vi "AlliGator Set New ROI Name.vi"(2 "Stored ROIs in":T1[](array[typedef]) {"ROI Descriptor"."Contours"."Type" items=["No Selection", "Point", "Line", "Rectangle", "Oval", "Polygon", "Freehand Region", "Annulus", "Unused2", "Unused3", "Broken Line", "Freehand Line", "Rotated Rectangle"]}, 3 "ROI Name in":string, 4 "Default Name (\"\")":string) -> (0 "ROI Name out":string)   [LabVIEW 2021, in "AlliGator ROIs.lvlib"]
doc: "Sets new ROI name (verifies that the input name is not already used)."
uses:
  Image/Named ROI Description.ctl
  AlliGator ROIs.lvlib
  Strings/Strings.lvlib
  Image/Image.lvlib
panel:
  # "see the AlliGator License on the block diagram (Ctrl+E or Window:Show Block Diagram)"
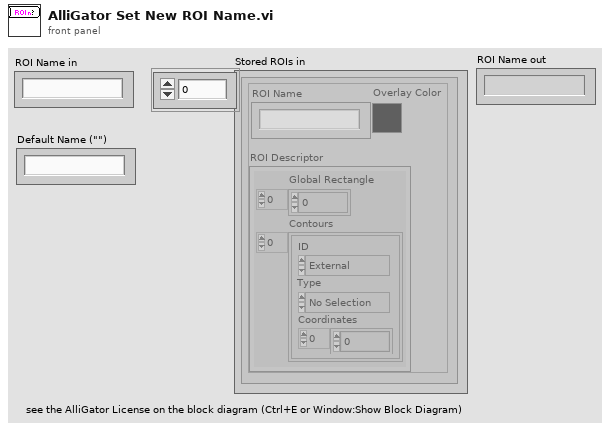
[diagram p1: front panel]
types:
  T1 = typedef "Image.lvlib/Named ROI Description.ctl" = cluster{"ROI Descriptor":T2, "ROI Name":string, "Overlay Color":u32}
  T2 = typedef "ROI Descriptor" = cluster{"Global Rectangle":i32[], "Contours":cluster{"ID":enum32{"External", "Internal"}, "Type":u32, "Coordinates":i32[]}[]}
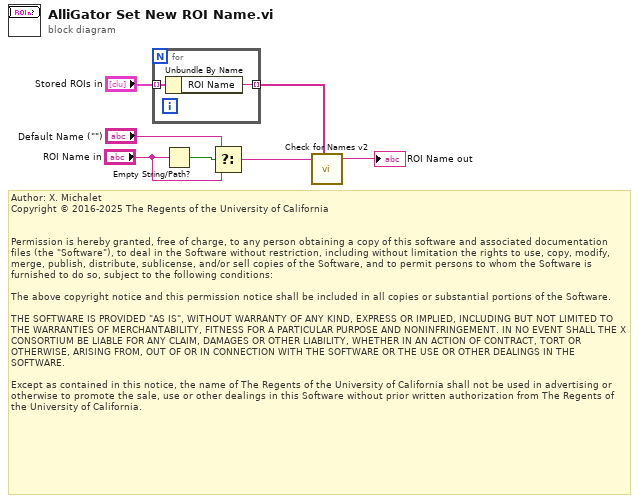
[diagram p0: block diagram]
diagram:
  # "Author: X. Michalet\nCopyright © 2016-2025 The Regents of the University of California\n \n\nPermission is hereby granted, free of charge, to any person obtaining a copy of this software and associated documentation files (the \"Software\"), to deal in the Software without restriction, including without limitation the rights to use, copy, modify, merge, publish, distribute, sublicense, and/or sell copies of the Software, and to permit persons to whom the Software is furnished to do so, subject to the following conditions:\n\nThe above copyright notice and this permission notice shall be included in all copies or substantial portions of the Software.\n\nTHE SOFTWARE IS PROVIDED \"AS IS\", WITHOUT WARRANTY OF ANY KIND, EXPRESS OR IMPLIED, INCLUDING BUT NOT LIMITED TO THE WARRANTIES OF MERCHANTABILITY, FITNESS FOR A PARTICULAR PURPOSE AND NONINFRINGEMENT. IN NO EVENT SHALL THE X CONSORTIUM BE LIABLE FOR ANY CLAIM, DAMAGES OR OTHER LIABILITY, WHETHER IN AN ACTION OF CONTRACT, TORT OR OTHERWISE, ARISING FROM, OUT OF OR IN CONNECTION WITH THE SOFTWARE OR THE USE OR OTHER DEALINGS IN THE SOFTWARE.\n\nExcept as contained in this notice, the name of The Regents of the University of California shall not be used in advertising or otherwise to promote the sale, use or other dealings in this Software without prior written authorization from The Regents of the University of California."
  n1 = for {
    tunnel: "Stored ROIs in" -> [w9] mode=indexing
    tunnel: [w8] -> w6 mode=indexing
    n2 = Unbundle By Name(w9) -> ("ROI Name"=w8:string)
  }
  n3 = Empty String/Path?(string/path="ROI Name in") -> (empty?=w4:bool)
  n4 = Select(t="Default Name (\"\")", s=w4, f="ROI Name in") -> (s? t:f=w1:string)
  n5 = call "Check for Names v2.vi"("New Name"=w1, "Name List"=w6) -> ("New Name"=→"ROI Name out":string)  [unwired: 4 in, 3 out]
